vi "Close.vi"(8 "error in (no error)":errorcluster, 11 "Fuji Delta in":refnum<class "Fuji Delta Robot.lvclass">) -> (0 "error out":errorcluster)   [LabVIEW 2014, in "Fuji Delta Robot.lvlib" / "Fuji Delta Robot.lvclass"]
uses:
  Fuji Delta Robot.lvclass
  Fuji Delta Robot.lvclass/Fuji Delta Robot.ctl
  ALPHA5 RS485/ALPHA5 RS485.lvlib
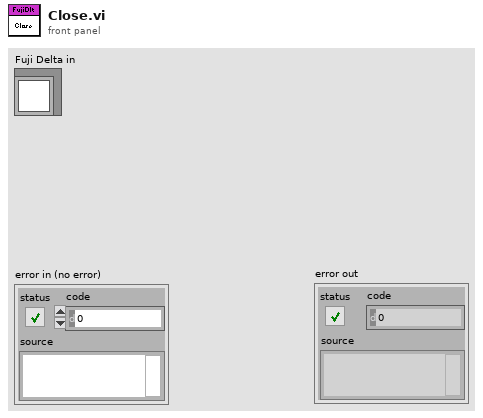
[diagram p1: front panel]
types:
  T1 = typedef "ALPHA5 RS485.lvlib/Port Selection Info.ctl" = cluster{"Port Name":refnum<visa-resource-name>, "Amplifier Num":u8, "Baud Rate":u32, "Char Formation":enum16{"0", "1", "2", "3", "4", "5"}}
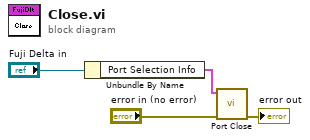
[diagram p0: block diagram]
diagram:
  n1 = Unbundle By Name("Fuji Delta in") -> ("Port Selection Info"=w3:T1)
  n2 = call "Port Close.vi"("error in (no error)"="error in (no error)", "Port Selection Info In"=w3) -> ("error out"=→"error out":errorcluster)  [unwired: 9 in]
